vi "doAction.vi"(8 "error in (no error)":errorcluster, 10 "ContextData":refnum<class "ContextData.lvclass">, 11 "Initialize in":refnum<class "Change Level.lvclass">) -> (0 "error out":errorcluster, 2 "ContextData Out":refnum<class "ContextData.lvclass">, 3 "Initialize out":refnum<class "Change Level.lvclass">)   [LabVIEW 2019, in "Change Level.lvclass"]
uses:
  Change Level.lvclass
  ContextData/ContextData.lvclass
  Change Level.lvclass/Change Level.ctl
  Simon_Engine/Simon_Engine.lvclass
  Messages/simonMessages/simonMessages.lvclass
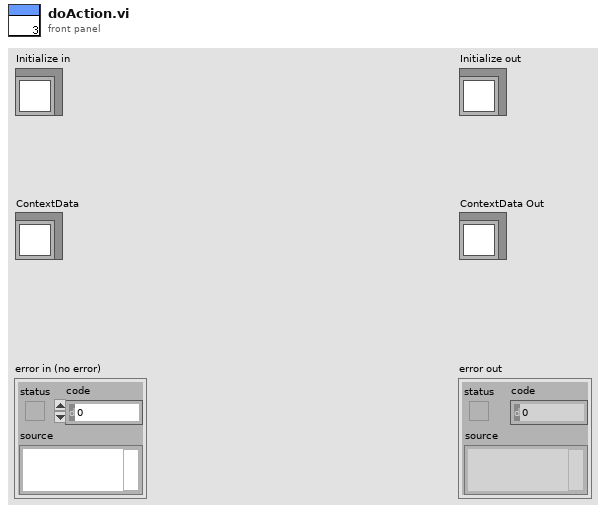
[diagram p1: front panel]
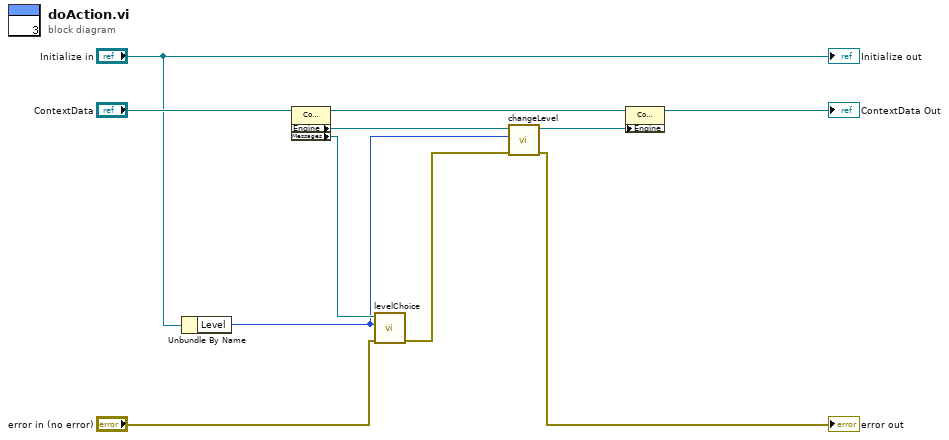
[diagram p0: block diagram]
diagram:
  n1 = Unbundle By Name("Initialize in") -> ("Level"=w1:u8)
  n2 = property class="ContextData.lvclass"(reference="ContextData") -> (reference out=w11:refnum<class "ContextData.lvclass">, "Engine"=w9:refnum<class "Simon_Engine.lvclass">, "Messages"=w7:refnum<class "simonMessages.lvclass">)  [unwired: 1 in, 1 out]
  n3 = call "levelChoice.vi"("error in (no error)"="error in (no error)", "Level Number"=w1, "simonMessages in"=w7) -> ("error out"=w10:errorcluster)  [unwired: 7 in, 1 out]
  n4 = call-dynamic "changeLevel.vi"("error in (no error)"=w10, "Level"=w1, "Simon_Engine in"=w9) -> ("error out"=→"error out":errorcluster, "Simon_Engine out"=w8:refnum<class "Simon_Engine.lvclass">)  [unwired: 7 in]
  n5 = property class="ContextData.lvclass"(reference=w11, "Engine"=w8) -> (reference out=→"ContextData Out":refnum<class "ContextData.lvclass">)  [unwired: 1 in, 1 out]
  "Initialize out" <- "Initialize in"
